vi "CPPpuff.vi"() -> ()   [LabVIEW 2022 SP3]
uses:
  Globals/Meas_global.vi
panel:
  out "totalTime":dbl=50000.0
  in  "PostPurge":dbl=25000.0
  in  "PulseGasChannel":i32=2
  in  "PurgeGasChannel":i32=1
  in  "WebPowerSwitch":string="10.245.69.7"
  in  "PrePurge":dbl=5000.0
  in  "Pulse":dbl=20000.0
  # "Trivial VI to pulse a pair of valves connected\nto a Web Power Switch, for FID response\ntesting                          TCRL 20210715"
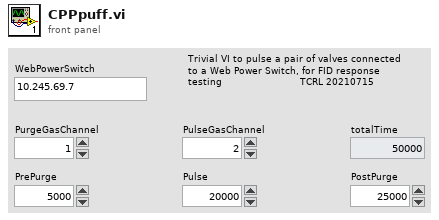
[diagram p1: front panel]
types:
  T1 = typedef "Post_Process.ctl" = enum16{"Take New Data", "Post Process Raw Data File"}
  T2 = typedef "Setup.ctl" = enum16{"Run Program", "Show Setup", "Save Current Setup", "Setup Front Panel"}
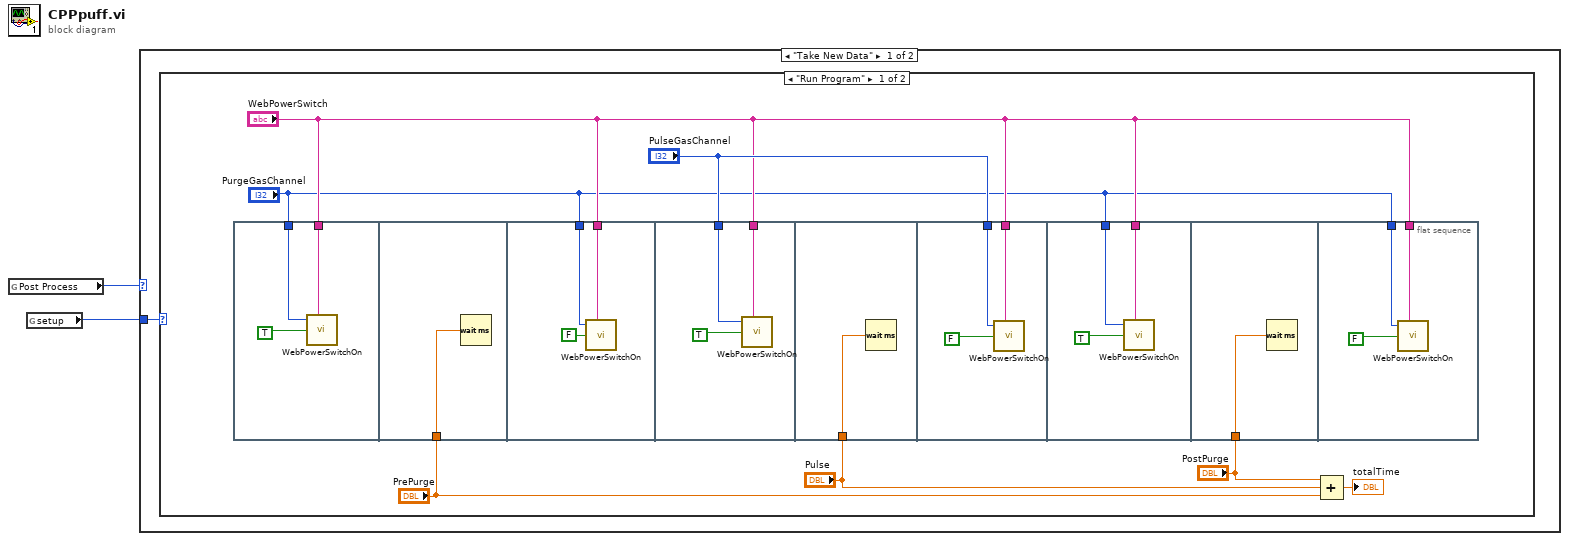
[diagram p0: block diagram]
diagram:
  n1 = global read "Meas_global.vi" "Post Process"() -> (w1:T1)
  n2 = global read "Meas_global.vi" "setup"() -> (w2:T2)
  n3 = case shown="\"Take New Data\"" w1 {
    tunnel: w2 -> [w3 _]
    frame "Take New Data" {
      n4 = case shown="\"Run Program\"" w3 {
        frame "Run Program" {
          n5 = flat-sequence {
            tunnel: "PurgeGasChannel" -> [w13]
            tunnel: "WebPowerSwitch" -> [w12]
            tunnel: "PrePurge" -> [w14]
            tunnel: "WebPowerSwitch" -> [w17]
            tunnel: "PurgeGasChannel" -> [w16]
            tunnel: "WebPowerSwitch" -> [w19]
            tunnel: "PulseGasChannel" -> [w18]
            tunnel: "Pulse" -> [w21]
            tunnel: "WebPowerSwitch" -> [w23]
            tunnel: "PulseGasChannel" -> [w22]
            tunnel: "WebPowerSwitch" -> [w26]
            tunnel: "PurgeGasChannel" -> [w25]
            tunnel: "PostPurge" -> [w28]
            tunnel: "WebPowerSwitch" -> [w30]
            tunnel: "PurgeGasChannel" -> [w29]
            frame #0 {
              n6 = call "WebPowerSwitchOn.vi"("WebPowerSwitchOutlet"=w13, "WebPowerSwitchIP"=w12, "DesiredState"=TRUE) -> ()  [unwired: 3 in, 2 out]
            }
            frame #1 {
              n7 = Wait (ms)(milliseconds to wait=w14) -> ()  [unwired: 1 out]
            }
            frame #2 {
              n8 = call "WebPowerSwitchOn.vi"("WebPowerSwitchOutlet"=w16, "WebPowerSwitchIP"=w17, "DesiredState"=FALSE) -> ()  [unwired: 3 in, 2 out]
            }
            frame #3 {
              n9 = call "WebPowerSwitchOn.vi"("WebPowerSwitchOutlet"=w18, "WebPowerSwitchIP"=w19, "DesiredState"=TRUE) -> ()  [unwired: 3 in, 2 out]
            }
            frame #4 {
              n10 = Wait (ms)(milliseconds to wait=w21) -> ()  [unwired: 1 out]
            }
            frame #5 {
              n11 = call "WebPowerSwitchOn.vi"("WebPowerSwitchOutlet"=w22, "WebPowerSwitchIP"=w23, "DesiredState"=FALSE) -> ()  [unwired: 3 in, 2 out]
            }
            frame #6 {
              n12 = call "WebPowerSwitchOn.vi"("WebPowerSwitchOutlet"=w25, "WebPowerSwitchIP"=w26, "DesiredState"=TRUE) -> ()  [unwired: 3 in, 2 out]
            }
            frame #7 {
              n13 = Wait (ms)(milliseconds to wait=w28) -> ()  [unwired: 1 out]
            }
            frame #8 {
              n14 = call "WebPowerSwitchOn.vi"("WebPowerSwitchOutlet"=w29, "WebPowerSwitchIP"=w30, "DesiredState"=FALSE) -> ()  [unwired: 3 in, 2 out]
            }
          }
          n15 = Compound Arithmetic op=ADD("PostPurge", "Pulse", "PrePurge") -> (→"totalTime":dbl)
        }
        frame "Show Setup", Default {
        }
      }
    }
    frame "Post Process Raw Data File", Default {
    }
  }
